vi "irradiance 1018_global variable.vi"() -> ()   [LabVIEW 2021]
panel:
  out "Irradiance ch 1018":dbl
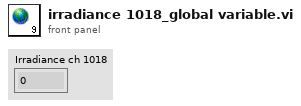
[diagram p1: front panel]
diagram:
